vi "ARINC 429 SEA Main Page.vi"(8 "error in (no error)":errorcluster, 11 "Node Ptr":T1 format="%.0x") -> (0 "error out":errorcluster)   [LabVIEW 2012, in "AIT 429 System Explorer.lvlib"]
uses:
  AIT 429 System Explorer.lvlib
  <vilib>/NI Veristand/Custom Device API/Custom Device Item Ref.ctl
  Shared/Controls and Global/Global.vi
  <vilib>/NI Veristand/Custom Device API/Get Item Property (Boolean).vi
  <vilib>/NI Veristand/Custom Device API/Get Item Property (Path).vi
  <vilib>/NI Veristand/Custom Device API/Get Item Property (String).vi
  <vilib>/NI Veristand/Custom Device API/Set Item Property (String).vi
  <vilib>/NI Veristand/Custom Device API/Custom Device API.lvlib
  Shared/ARINC 429 Shared.lvlib
  <vilib>/NI Veristand/Custom Device API/Set Item Property (Boolean).vi
panel:
  out "Version":string
  in  "ScheduledSDI?":bool
  in  "RefreshDB":bool
  in  "Warning text":string="WARNING: The database has changed since import. If you attempt to run this system definition an error may occur. Consider refreshing the database import."
  out "Warn Icon":bool
  out "Database File":path
  in  "Header":cluster{"Section Name":string}={"Section Name"="ARINC 429 - SEA -  Custom Device"}
  in  "Description":string
  in  "Name":string
  # "SEA 9811 module configuration is hardcoded in the RT Driver VI"
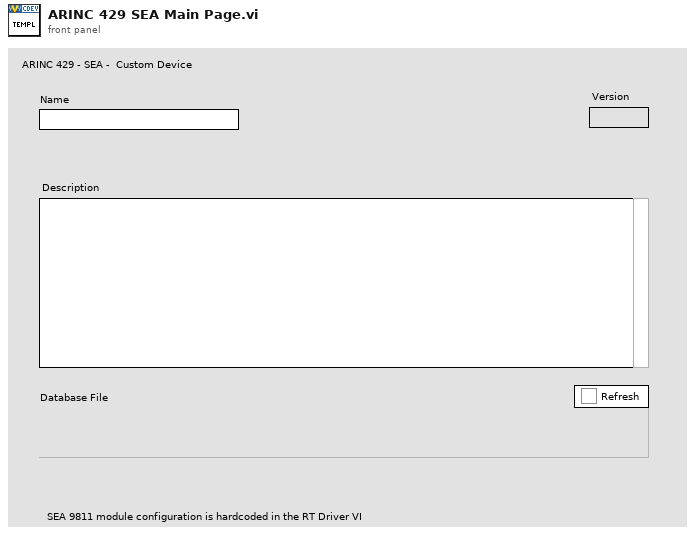
[diagram p1: front panel]
types:
  T1 = typedef "Custom Device API.lvlib/Custom Device Item Ref.ctl" = u64
  T2 = typedef "Custom Device API.lvlib/Custom Device Item Info.ctl" = cluster{"Name":string, "Is Channel":bool, "GUID":string, "Is Waveform":bool}
  T3 = typedef "Custom Device API.lvlib/Custom Device Commands.ctl" = enum16{"Default", "Item renamed", "Shutdown", "Dynamic button pressed"}
  T4 = typedef "AIT 429 System Explorer.lvlib/Refresh Match Settings.ctl" = cluster{"Ch by name?":bool, "Lbl by name?":bool}
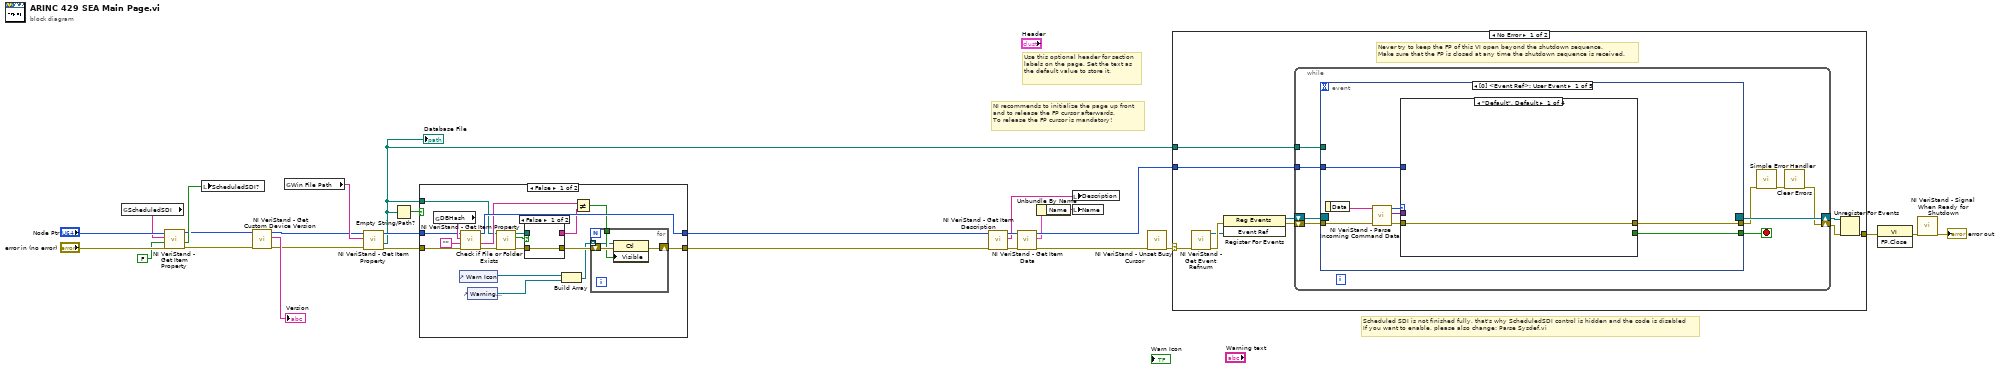
[diagram p0: block diagram]
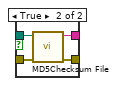
[diagram p2: hidden frame]
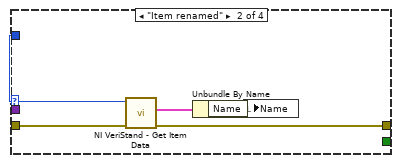
[diagram p4: hidden frame]
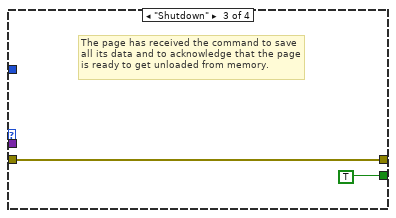
[diagram p5: hidden frame]
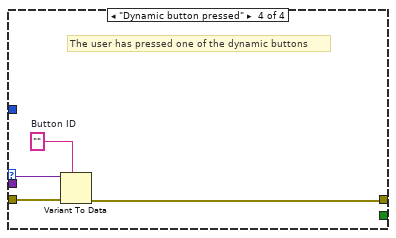
[diagram p6: hidden frame]
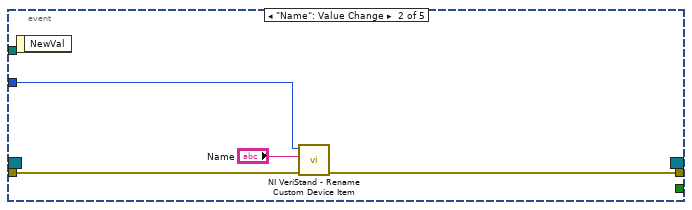
[diagram p7: hidden frame]
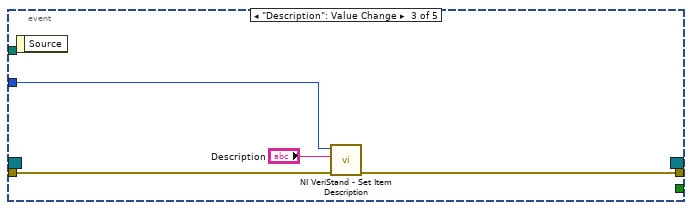
[diagram p8: hidden frame]
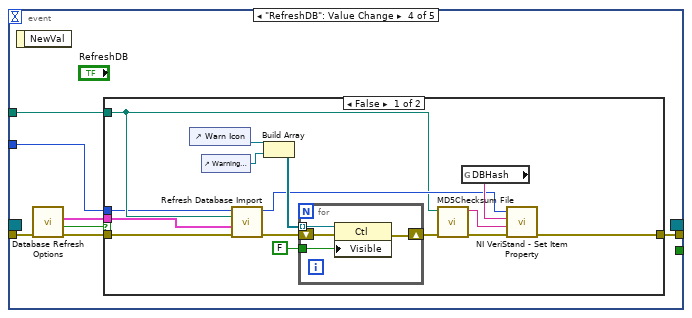
[diagram p9: hidden frame]
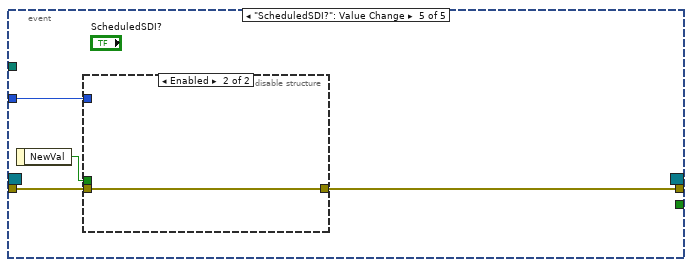
[diagram p11: hidden frame]
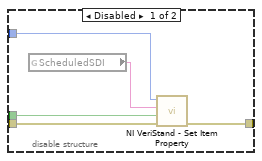
[diagram p12: hidden frame]
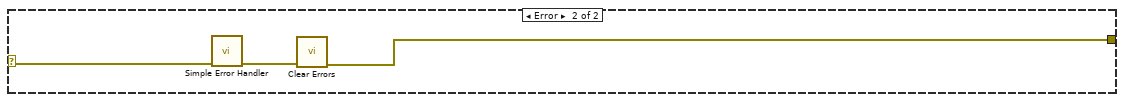
[diagram p13: hidden frame]
diagram:
  # "Scheduled SDI is not finished fully, that's why ScheduledSDI control is hidden and the code is disabled\nIf you want to enable, please also change: Parse Sysdef.vi"
  # "Use this optional header for section labels on the page. Set the text as the default value to store it."
  # "NI recommends to initialize the page up front\nand to release the FP cursor afterwards.\nTo release the FP cursor is mandatory!"
  n1 = global read "Global.vi" "ScheduledSDI"() -> (w7:string)
  n2 = call-poly <vilib>:"NI VeriStand - Get Item Property.vi"("error in (no error)"="error in (no error)", "Default Value"=FALSE, "Property Name"=w7, "Item Ref in"="Node Ptr") -> ("error out"=w8:errorcluster, "Value"=w5:bool, "Item Ref out"=w4:T1)  [unwired: 4 in, 1 out]
  n3 = local write "ScheduledSDI?"(w5) -> ()
  n4 = call <vilib>:"NI VeriStand - Get Custom Device Version.vi"("error in (no error)"=w8, "Device Ref in"=w4) -> ("error out"=w1:errorcluster, "Value"=→"Version":string, "Device Ref out"=w2:T1)  [unwired: 7 in]
  n5 = global read "Global.vi" "Win File Path"() -> (w17:string)
  n6 = call-poly <vilib>:"NI VeriStand - Get Item Property.vi"("error in (no error)"=w1, "Property Name"=w17, "Item Ref in"=w2) -> ("error out"=w15:errorcluster, "Value"=w11:path, "Item Ref out"=w12:T1)  [unwired: 5 in, 1 out]
  "Database File" <- w11
  n7 = Empty String/Path?(string/path=w11) -> (empty?=w16:bool)
  n8 = case shown="False" w16 {
    tunnel: w15 -> [w43 w57]
    tunnel: [w34 w57] -> w14
    tunnel: [w42 w56] -> w13
    tunnel: w12 -> [w44 w56]
    tunnel: w11 -> [w30 _]
    frame False {
      n9 = global read "Global.vi" "DBHash"() -> (w45:string)
      n10 = control-ref of="Warn Icon"() -> (w36:refnum<vi>)
      n11 = call-poly <vilib>:"NI VeriStand - Get Item Property.vi"("error in (no error)"=w43, "Default Value"="", "Property Name"=w45, "Item Ref in"=w44) -> ("error out"=w31:errorcluster, "Value"=w40:string, "Item Ref out"=w42:T1)  [unwired: 4 in, 1 out]
      n12 = control-ref of="Warning text"() -> (w37:refnum<vi>)
      n13 = call <vilib>:"Check if File or Folder Exists.vi"("error in (no error)"=w31, "path"=w30) -> ("error out"=w33:errorcluster, "file or folder exists?"=w29:bool, "dup path"=w32:path)  [unwired: 7 in]
      n14 = case shown="False" w29 {
        tunnel: [_ w51] -> w41
        tunnel: [w47 w50] -> w39
        tunnel: w33 -> [w47 w49]
        tunnel: w32 -> [_ w48]
        frame False {
        }
        frame True {
          n15 = call <vilib>:"MD5Checksum File.vi"("error in (no error)"=w49, "Path"=w48) -> ("error out"=w50:errorcluster, "MD5 message-digest"=w51:string)  [unwired: 8 in]
        }
      }
      n16 = Build Array(w36, w37) -> (w35:refnum<vi>[])
      n17 = Not Equal?(x=w40, y=w41) -> (x != y?=w38:bool)
      n18 = for {
        shift-right: [w54] -> w34
        shift-left: w39 -> [w55]
        tunnel: w38 -> [w53]
        tunnel: w35 -> [w52] mode=indexing
        n19 = property class="Ctl"(reference=w52, error in=w55, "Visible"=w53) -> (error out=w54:errorcluster)  [unwired: 1 out]
      }
    }
    frame True {
    }
  }
  n20 = call <vilib>:"NI VeriStand - Get Item Description.vi"("error in (no error)"=w14, "Item Ref in"=w13) -> ("error out"=w20:errorcluster, "Description"=w21:string, "Item Ref out"=w22:T1)  [unwired: 7 out]
  n21 = call <vilib>:"NI VeriStand - Get Item Data.vi"("error in (no error)"=w20, "Item Ref in"=w22) -> ("error out"=w25:errorcluster, "Item Info"=w19:T2, "Item Ref out"=w23:T1)  [unwired: 7 out]
  n22 = Unbundle By Name(w19) -> ("Name"=w18:string)
  n23 = local write "Description"(w21) -> ()
  n24 = local write "Name"(w18) -> ()
  n25 = call <vilib>:"NI VeriStand - Unset Busy Cursor.vi"("error in (no error)"=w25) -> ("error out"=w24:errorcluster)  [unwired: 10 out]
  n26 = case shown="No Error" w24 {
    selector: w24 -> [w59 w144]
    tunnel: [w64 w142] -> w28
    tunnel: w23 -> [w60 _]
    tunnel: w11 -> [w58 _]
    frame No Error {
      # "Never try to keep the FP of this VI open beyond the shutdown sequence.\nMake sure that the FP is closed at any time the shutdown sequence is received."
      n27 = call <vilib>:"NI VeriStand - Get Event Refnum.vi"("error in (no error)"=w59) -> ("error out"=w67:errorcluster, "Event Ref"=w63:refnum<user-event>)  [unwired: 9 out]
      n28 = register-events(error in=w67, w63) -> (reference out=w61:refnum<event-registration>, error out=w62:errorcluster)  [unwired: 1 in]
      n29 = while {
        tunnel: w60 -> [w72]
        shift-right: [w69] -> w65
        shift-left: w62 -> [w75]
        shift-right: [w76] -> w66
        shift-left: w61 -> [w74]
        tunnel: w58 -> [w68]
        stop <- w73 stop-if-true
        n30 = event shown="[0] <Event Ref>: User Event" {
          selector: w74 -> [_ _ _ _ _]
          dyn-events: [_ _ _ _ _] -> w76
          timeout: _ -> [_ _ _ _ _]
          tunnel: w75 -> [w84 w100 w103 w106 w135]
          tunnel: [w80 _ _ _ _] -> w73
          tunnel: [w79 w99 w102 w105 w132] -> w71
          tunnel: w72 -> [w78 w98 w104 w110 w134]
          tunnel: w68 -> [_ _ _ w111 _]
          event User Event {
            n31 = event-data() -> ("Data"=w83:string)  [unwired: 1 out]
            n32 = call <vilib>:"NI VeriStand - Parse Incoming Command Data.vi"("error in (no error)"=w84, "Incoming data"=w83) -> ("error out"=w82:errorcluster, "Outgoing data"=w77:variant, "Action"=w81:T3)  [unwired: 7 out]
            n33 = case shown="\"Default\", Default" w81 {
              tunnel: w82 -> [w85 w90 w91 w96]
              tunnel: [_ _ TRUE _] -> w80
              tunnel: [w85 w87 w91 w93] -> w79
              tunnel: w78 -> [_ w89 _ _]
              tunnel: w77 -> [_ _ _ w95]
              frame "Default", Default {
              }
              frame "Item renamed" {
                n34 = call <vilib>:"NI VeriStand - Get Item Data.vi"("error in (no error)"=w90, "Item Ref in"=w89) -> ("error out"=w87:errorcluster, "Item Info"=w88:T2)  [unwired: 8 out]
                n35 = Unbundle By Name(w88) -> ("Name"=w86:string)
                n36 = local write "Name"(w86) -> ()
              }
              frame "Shutdown" {
                # "The page has received the command to save all its data and to acknowledge that the page is ready to get unloaded from memory."
              }
              frame "Dynamic button pressed" {
                w94 = ""  # Button ID
                # "The user has pressed one of the dynamic buttons"
                n37 = Variant To Data(error in=w96, type=w94, Variant=w95) -> (error out=w93:errorcluster)  [unwired: 1 out]
              }
            }
          }
          event "Name": Value Change {
            n38 = event-data() -> ()  [unwired: 2 out]
            n39 = call <vilib>:"NI VeriStand - Rename Custom Device Item.vi"("error in (no error)"=w100, "New Name"="Name", "Item Ref in"=w98) -> ("error out"=w99:errorcluster)  [unwired: 1 in, 7 out]
          }
          event "Description": Value Change {
            n40 = event-data() -> ()  [unwired: 2 out]
            n41 = call <vilib>:"NI VeriStand - Set Item Description.vi"("error in (no error)"=w103, "Description"="Description", "Item Ref in"=w104) -> ("error out"=w102:errorcluster)  [unwired: 8 out]
          }
          event "RefreshDB": Value Change {
            n42 = event-data() -> ()  [unwired: 2 out]
            n43 = call "Database Refresh Options.vi"("error in (no error)"=w106) -> ("error out"=w109:errorcluster, "Cancelled?"=w108:bool, "Refresh Settings"=w107:T4)  [unwired: 8 in]
            n44 = case shown="False" w108 {
              tunnel: [w113 w131] -> w105
              tunnel: w109 -> [w112 w131]
              tunnel: w111 -> [w116 _]
              tunnel: w110 -> [w115 _]
              tunnel: w107 -> [w114 _]
              frame False {
                n45 = control-ref of="Warn Icon"() -> (w122:refnum<vi>)
                n46 = control-ref of="Warning text"() -> (w123:refnum<vi>)
                n47 = call "Refresh Database Import.vi"("error in (no error)"=w112, "Match settings"=w114, "DB"=w116, "Item Ref in"=w115) -> ("error out"=w118:errorcluster, "Item Ref dup"=w117:T1)  [unwired: 5 in, 1 out]
                n48 = Build Array(w122, w123) -> (w120:refnum<vi>[])
                n49 = for {
                  shift-right: [w129] -> w121
                  shift-left: w118 -> [w130]
                  tunnel: w120 -> [w128] mode=indexing
                  tunnel: FALSE ("Visible") -> [w127]
                  n50 = property class="Ctl"(reference=w128, error in=w130, "Visible"=w127) -> (error out=w129:errorcluster)  [unwired: 1 out]
                }
                n51 = call <vilib>:"MD5Checksum File.vi"("error in (no error)"=w121, "Path"=w116) -> ("error out"=w126:errorcluster, "MD5 message-digest"=w125:string)  [unwired: 8 in]
                n52 = global read "Global.vi" "DBHash"() -> (w124:string)
                n53 = call-poly <vilib>:"NI VeriStand - Set Item Property.vi"("error in (no error)"=w126, "Value"=w125, "Property Name"=w124, "Item Ref in"=w117) -> ("error out"=w113:errorcluster)  [unwired: 5 in, 2 out]
              }
              frame True {
              }
            }
          }
          event "ScheduledSDI?": Value Change {
            n54 = event-data() -> ("NewVal"=w133:bool)  [unwired: 1 out]
            n55 = disable-structure shown="Enabled" {
              disable-tunnel: w135 -> [w140 w141]
              disable-tunnel: w134 -> [w139 _]
              disable-tunnel: w133 -> [w138 _]
              disable-tunnel: [w137 w141] -> w132
              frame Disabled {
                n56 = global read "Global.vi" "ScheduledSDI"() -> (w136:string)
                n57 = call-poly <vilib>:"NI VeriStand - Set Item Property.vi"("error in (no error)"=w140, "Value"=w138, "Property Name"=w136, "Item Ref in"=w139) -> ("error out"=w137:errorcluster)  [unwired: 5 in, 2 out]
              }
              frame Enabled {
              }
            }
          }
        }
        n58 = call <vilib>:"Simple Error Handler.vi"("error in (no error)"=w71) -> ("error out"=w70:errorcluster)  [unwired: 1 in, 7 out]
        n59 = call <vilib>:"Clear Errors.vi"("error in (no error)"=w70) -> ("error out"=w69:errorcluster)  [unwired: 6 out]
      }
      n60 = Unregister For Events(event registration refnum=w66, error in=w65) -> (error out=w64:errorcluster)
    }
    frame Error {
      n61 = call <vilib>:"Simple Error Handler.vi"("error in (no error)"=w144) -> ("error out"=w143:errorcluster)  [unwired: 1 in, 7 out]
      n62 = call <vilib>:"Clear Errors.vi"("error in (no error)"=w143) -> ("error out"=w142:errorcluster)  [unwired: 6 out]
    }
  }
  n63 = invoke class="VI" method="FP.Close"(error in=w28) -> (error out=w27:errorcluster)  [unwired: 2 in, 2 out]
  n64 = call <vilib>:"NI VeriStand - Signal When Ready for Shutdown.vi"("error in (no error)"=w27) -> ("error out"=→"error out":errorcluster)  [unwired: 10 out]
